vi "Switch Protection Signal For Auto.vi"(8 "error in (no error)":errorcluster, 9 "Protected Signal GUID":string, 10 "Protection Value GUID":string, 11 "Node Ptr":T1 format="%.0x") -> (0 "error out":errorcluster)   [LabVIEW 2023, in "Protection and Counter Support System Explorer.lvlib"]
uses:
  Protection and Counter Support System Explorer.lvlib
  <vilib>/NI VeriStand/Custom Device API/Custom Device Item Ref.ctl
  <vilib>/NI VeriStand/Custom Device API/Custom Device API.lvlib
  Types/Protection Signal Linked Channel.ctl
  Shared/Types/Protection Type.ctl
  Shared/Protection and Counter Support Shared.lvlib
  Types/Protection Signal Settings.ctl
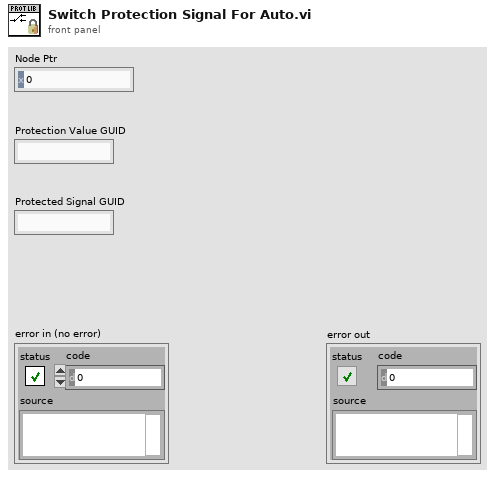
[diagram p1: front panel]
types:
  T1 = typedef "Custom Device API.lvlib/Custom Device Item Ref.ctl" = u64
  T2 = typedef "Protection and Counter Support Shared.lvlib/Protection Type.ctl" = enum16{"Arb ID + Bytes Checksum with Inversion", "Arb ID + Bytes CRC with Inversion", "Reversed Raw Signal Checksum with Inversion", "Concatenated Two's Compliment", "LP_CRC8"}
  T3 = typedef "Protection and Counter Support System Explorer.lvlib/Protection Signal Settings.ctl" = cluster{"Input Channels":T4[], "Protection Type":T2}
  T4 = typedef "Protection and Counter Support System Explorer.lvlib/Protection Signal Linked Channel.ctl" = cluster{"Node Ref":T1}
  T5 = typedef "Custom Device API.lvlib/Custom Device Item Info.ctl" = cluster{"Name":string, "Is Channel":bool, "GUID":string, "Is Waveform":bool}
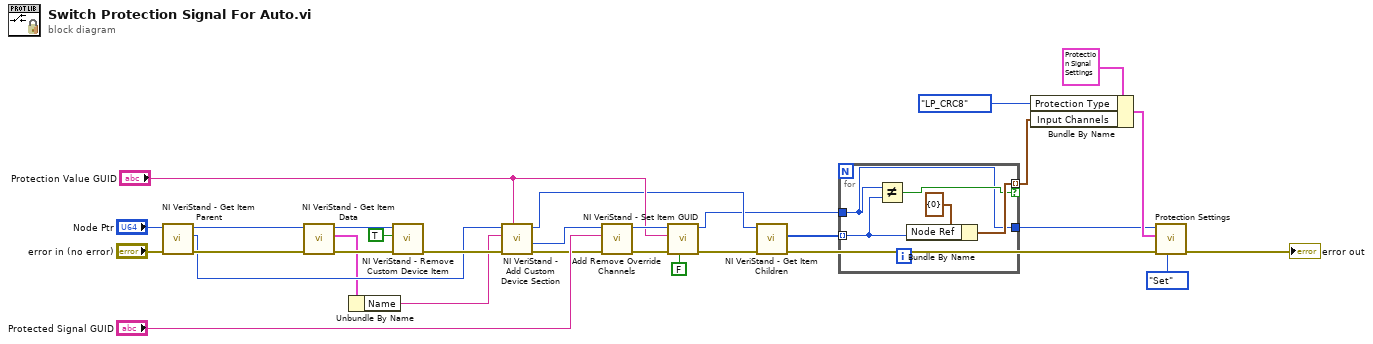
[diagram p0: block diagram]
diagram:
  n1 = call <vilib>:"NI VeriStand - Get Item Parent.vi"("error in (no error)"="error in (no error)", "Item Ref in"="Node Ptr") -> ("error out"=w23:errorcluster, "Parent Ref"=w21:T1, "Item Ref out"=w25:T1)  [unwired: 6 in, 1 out]
  n2 = call <vilib>:"NI VeriStand - Get Item Data.vi"("error in (no error)"=w23, "Item Ref in"=w25) -> ("error out"=w19:errorcluster, "Item Info"=w18:T5, "Item Ref out"=w20:T1)  [unwired: 6 in, 1 out]
  n3 = Unbundle By Name(w18) -> ("Name"=w17:string)
  n4 = call <vilib>:"NI VeriStand - Remove Custom Device Item.vi"("error in (no error)"=w19, "Force Delete (F)"=TRUE, "Item Ref in"=w20) -> ("error out"=w22:errorcluster)  [unwired: 7 in, 1 out]
  n5 = call <vilib>:"NI VeriStand - Add Custom Device Section.vi"("GUID (Default Section)"="Protection Value GUID", "error in (no error)"=w22, "Section Name"=w17, "Parent Ref in"=w21) -> ("error out"=w14:errorcluster, "Section Ptr"=w15:T1, "Parent Ref out"=w5:T1)  [unwired: 4 in, 1 out]
  n6 = call "Add Remove Override Channels.vi"("error in (no error)"=w14, "Protected Signal GUID"="Protected Signal GUID", "Channel Ref in"=w15) -> ("error out"=w29:errorcluster, "Channel Ref out"=w30:T1)  [unwired: 7 in]
  n7 = call <vilib>:"NI VeriStand - Set Item GUID.vi"("Refresh System Explorer Tree? (F)"=FALSE, "error in (no error)"=w29, "GUID"="Protection Value GUID", "Item Ref in"=w30) -> ("error out"=w7:errorcluster, "Item Ref out"=w2:T1)  [unwired: 6 in]
  n8 = call <vilib>:"NI VeriStand - Get Item Children.vi"("error in (no error)"=w7, "Item Ref in"=w5) -> ("error out"=w6:errorcluster, "Child Refs"=w4:T1[])  [unwired: 6 in, 2 out]
  n9 = for {
    tunnel: w4 -> [w33] mode=indexing
    tunnel: [w34] -> w3 mode=indexing if=w32
    tunnel: w2 -> [w31]
    tunnel: [w31] -> w1
    n10 = Not Equal?(x=w31, y=w33) -> (x != y?=w32:bool)
    n11 = Bundle By Name(cluster=T4 {"Node Ref"=0} ("MonitoredChannelSettings"), "Node Ref"=w33) -> (w34:T4)
  }
  n12 = Bundle By Name(cluster=T3 {"Input Channels"=[], "Protection Type"=enum."Arb ID + Bytes Checksum with Inversion"} ("Selected Channels"), "Protection Type"=Protection_Type."LP_CRC8", "Input Channels"=w3) -> (w8:T3)
  n13 = call "Protection Settings.vi"("Action"=enum8{"Get", "Set"}."Set", "error in"=w6, "Selected Channels"=w8, "Parent Ref"=w1) -> ("error out"=→"error out":errorcluster)  [unwired: 5 in, 2 out]
